vi "LoadAllPodsData.vi"(10 "Configuration Data in":T1, 11 "Config file Refnum in":T2) -> (2 "Configuration Data out":T1, 3 "Config fileRefnum out":T2)   [LabVIEW 2014]
uses:
  <vilib>/Utility/config.llb/Config Data RefNum.ctl
  Variables/References.vi
  <vilib>/Utility/config.llb/NI_LVConfig.lvlib
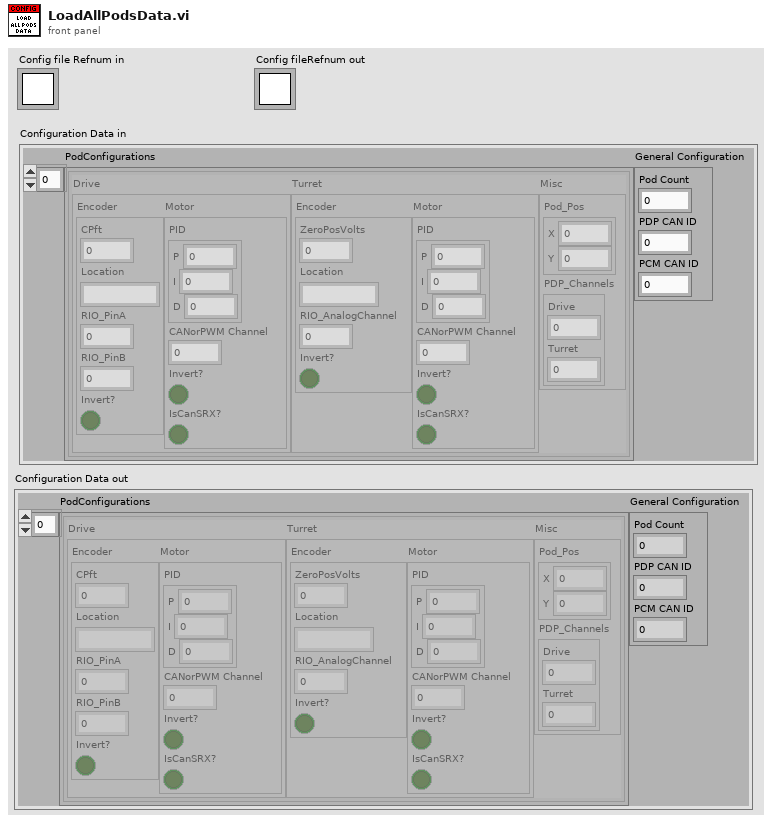
[diagram p1: front panel]
types:
  T1 = cluster{"PodConfigurations":cluster{"Drive":cluster{"Encoder":cluster{"CPft":dbl, "Location":string, "RIO_PinA":i32, "RIO_PinB":i32, "Invert?":bool}, "Motor":cluster{"PID":cluster{"P":dbl, "I":dbl, "D":dbl}, "CANorPWM Channel":i32, "Invert?":bool, "IsCanSRX?":bool}}, "Turret":cluster{"Encoder":cluster{"ZeroPosVolts":dbl, "Location":string, "RIO_AnalogChannel":i32, "Invert?":bool}, "Motor":cluster{"PID":cluster{"P":dbl, "I":dbl, "D":dbl}, "CANorPWM Channel":i32, "Invert?":bool, "IsCanSRX?":bool}}, "Misc":cluster{"Pod_Pos":cluster{"X":dbl, "Y":dbl}, "PDP_Channels":cluster{"Drive":i32, "Turret":i32}}}[], "General Configuration":cluster{"Pod Count":i32, "PDP CAN ID":i32, "PCM CAN ID":i32}}
  T2 = typedef "NI_LVConfig.lvlib/Config Data RefNum.ctl" = refnum<k1>
  T3 = cluster{"Drive":cluster{"Encoder":cluster{"CPft":dbl, "Location":string, "RIO_PinA":i32, "RIO_PinB":i32, "Invert?":bool}, "Motor":cluster{"PID":cluster{"P":dbl, "I":dbl, "D":dbl}, "CANorPWM Channel":i32, "Invert?":bool, "IsCanSRX?":bool}}, "Turret":cluster{"Encoder":cluster{"ZeroPosVolts":dbl, "Location":string, "RIO_AnalogChannel":i32, "Invert?":bool}, "Motor":cluster{"PID":cluster{"P":dbl, "I":dbl, "D":dbl}, "CANorPWM Channel":i32, "Invert?":bool, "IsCanSRX?":bool}}, "Misc":cluster{"Pod_Pos":cluster{"X":dbl, "Y":dbl}, "PDP_Channels":cluster{"Drive":i32, "Turret":i32}}}[]
  T4 = cluster{"Drive":cluster{"Encoder":cluster{"CPft":dbl, "Location":string, "RIO_PinA":i32, "RIO_PinB":i32, "Invert?":bool}, "Motor":cluster{"PID":cluster{"P":dbl, "I":dbl, "D":dbl}, "CANorPWM Channel":i32, "Invert?":bool, "IsCanSRX?":bool}}, "Turret":cluster{"Encoder":cluster{"ZeroPosVolts":dbl, "Location":string, "RIO_AnalogChannel":i32, "Invert?":bool}, "Motor":cluster{"PID":cluster{"P":dbl, "I":dbl, "D":dbl}, "CANorPWM Channel":i32, "Invert?":bool, "IsCanSRX?":bool}}, "Misc":cluster{"Pod_Pos":cluster{"X":dbl, "Y":dbl}, "PDP_Channels":cluster{"Drive":i32, "Turret":i32}}}
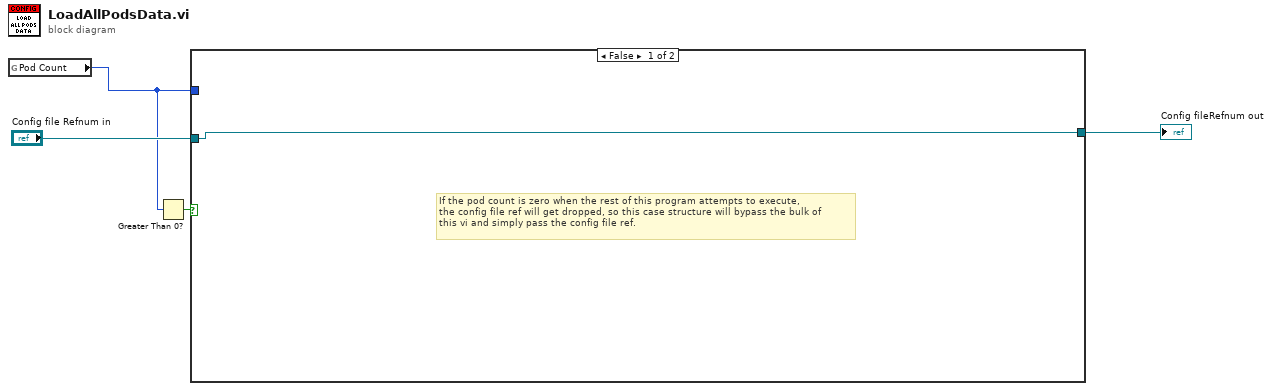
[diagram p0: block diagram]
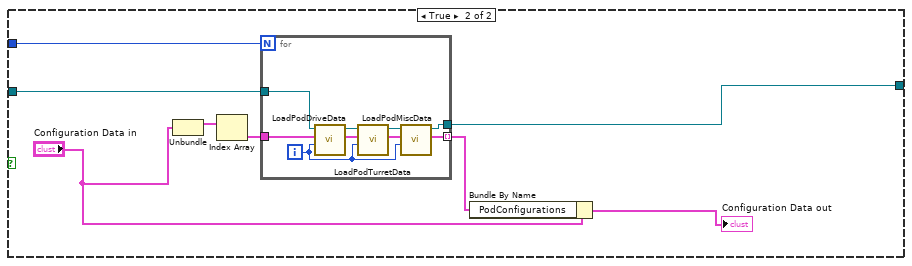
[diagram p2: hidden frame]
diagram:
  n1 = global read "References.vi" "Pod Count"() -> (w1:i32)
  n2 = Greater Than 0?(x=w1) -> (x > 0?=w2:bool)
  n3 = case shown="False" w2 {
    tunnel: [w5 w13] -> w4
    tunnel: "Config file Refnum in" -> [w5 w12]
    tunnel: w1 -> [_ w8]
    frame False {
      # "If the pod count is zero when the rest of this program attempts to execute,\nthe config file ref will get dropped, so this case structure will bypass the bulk of\nthis vi and simply pass the config file ref."
    }
    frame True {
      n4 = Unbundle("Configuration Data in") -> ("PodConfigurations"=w10:T3)  [unwired: 1 out]
      n5 = Index Array(array=w10) -> (element=w11:T4)  [unwired: 1 in]
      n6 = for {
        N: w8 -> [_]
        tunnel: w11 -> [w22]
        tunnel: w12 -> [w21]
        tunnel: [w14] -> w13
        tunnel: [w15] -> w9 mode=indexing
        i -> [w17]
        n7 = call "LoadPodDriveData.vi"("Pod Number"=w17, "Pod Configuration in"=w22, "Config file Refnum in"=w21) -> ("Pod Configuration out"=w20:T4, "Config file Refnum out"=w19:T2)  [unwired: 7 in]
        n8 = call "LoadPodTurretData.vi"("Pod Number"=w17, "Pod Configuration in"=w20, "Config file Refnum in"=w19) -> ("Pod Configuration out"=w18:T4, "Config file Refnum out"=w16:T2)  [unwired: 7 in]
        n9 = call "LoadPodMiscData.vi"("Pod Number"=w17, "Pod Configuration in"=w18, "Config File Refnum in"=w16) -> ("Pod Configuration out"=w15:T4, "Config File Refnum out"=w14:T2)  [unwired: 7 in]
      }
      n10 = Bundle By Name(cluster="Configuration Data in", "PodConfigurations"=w9) -> (→"Configuration Data out":T1)
    }
  }
  "Config fileRefnum out" <- w4
